vi "scope.vi"(7 "Channel Name":string="0" caption="Channel(s)", 8 "Trigger Type":T1(tab)=enum."Hysteresis", 9 "Min Sample Rate":dbl=10000.0 caption="Min. Sample Rate" step=1000000.0 format="%#.2p", 10 "error in":errorcluster, 11 "instrument handle":refnum<k15>) -> (0 "median":dbl=-0.00010879155888687819 format="%0.2f", 1 "Waveform(s)":waveform(dbl)(graph), 2 "error out":errorcluster, 3 "instrument handle out":refnum<k15>, 4 "low_level":dbl=-0.00010879155888687819, 6 "high_level":dbl=0.016276325847857098)   [LabVIEW 2018]
uses:
  <instrlib>/niScope/Configure/Trigger/niScope Configure Trigger Immediate.vi
  <instrlib>/niScope/Configure/Trigger/niScope Configure Trigger Edge.vi
  <instrlib>/niScope/Configure/Trigger/niScope Configure Trigger Digital.vi
  <instrlib>/niScope/Configure/Trigger/niScope Configure Trigger Window.vi
  <instrlib>/niScope/Configure/Trigger/niScope Configure Trigger Hysteresis.vi
  <instrlib>/niScope/Acquire/Fetch/niScope Fetch WDT.vi
  <vilib>/Analysis/NI_AALBase.lvlib
panel:
  in  "Trigger Source":string(combo)="0"
  in  "Trigger Level":dbl format="%.2f"
  in  "Trigger Slope":i32(ring) items=["Positive", "Negative"]
  in  "Coupling":u16(ring)=1 caption="Trigger Coupling" items=["AC"=0, "DC"=1, "HF Reject"=3, "LF Reject"=4, "AC Plus HF Reject"=1001]
  in  "Trigger Slope 2":i32(ring) caption="Trigger Slope" items=["Positive", "Negative"]
  in  "Trigger Source 2":string(combo)="VAL_PFI_1" caption="Trigger Source"
  in  "Coupling 2":u16(ring)=1 caption="Trigger Coupling" items=["AC"=0, "DC"=1, "HF Reject"=3, "LF Reject"=4, "AC Plus HF Reject"=1001]
  in  "High Level":dbl=0.1 caption="Window High Level" format="%.2f"
  in  "Low Level":dbl=-0.1 caption="Window Low Level" format="%.2f"
  in  "Window Mode":i32(ring) items=["Entering", "Leaving"]
  in  "Trigger Source 3":string(combo)="0" caption="Trigger Source"
  in  "Hysteresis":dbl=0.05 format="%.2f"
  in  "Trigger Source 4":string(combo)="0" caption="Trigger Source"
  in  "Trigger Level 2":dbl caption="Trigger Level" format="%.2f"
  in  "Coupling 3":u16(ring)=1 caption="Trigger Coupling" items=["AC"=0, "DC"=1, "HF Reject"=3, "LF Reject"=4, "AC Plus HF Reject"=1001]
  in  "Trigger Slope 3":i32(ring) caption="Trigger Slope" items=["Positive", "Negative"]
  out "Auto Triggered":bool=TRUE
  in  "Trigger Modifier":i32(ring)=2 items=["None"=1, "Auto Trigger"=2]
  in  "Vertical Coupling":i32(ring)=1 items=["AC", "DC", "Ground"]
  in  "Reference Position":dbl=50.0 caption="Ref Position" format="%.1f"
  in  "Trigger Delay":dbl caption="Trigger Delay (s)" format="%#.4p"
  in  "Maximum Input Frequency":dbl caption="Max. Input Frequency (Hz)" format="%.2f"
  in  "Input Impedance":u32(ring) items=["1 mega ohm"=0, "50 ohms"=2]
  in  "Probe Attenuation":dbl=1.0 format="%.1f"
  in  "Vertical Offset":dbl caption="Vertical Offset (V)" format="%.2p"
  in  "Timeout (s)":dbl=5.0 caption="Timeout(s)" format="%.2f"
  out "Actual Sample Rate":dbl=10000.0 format="%#.2p"
  out "Actual Record Length":i32=500
  in  "Min Record Length":i32=1000 caption="Min. Record Length"
  in  "Vertical Range":dbl=4.0 caption="Vertical Range (V)" format="%.2f"
  in  "Enforce Realtime":bool=TRUE
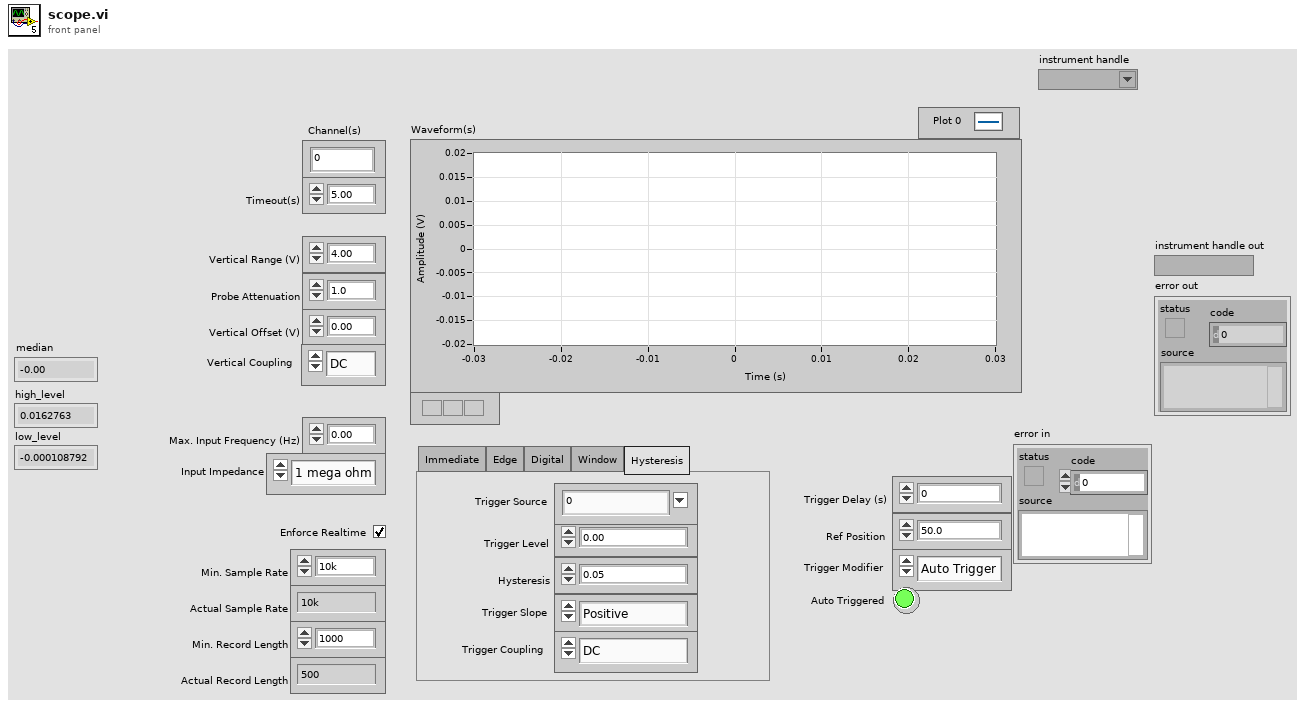
[diagram p1: front panel]
types:
  T1 = enum32{"Immediate", "Edge", "Digital", "Window", "Hysteresis"}
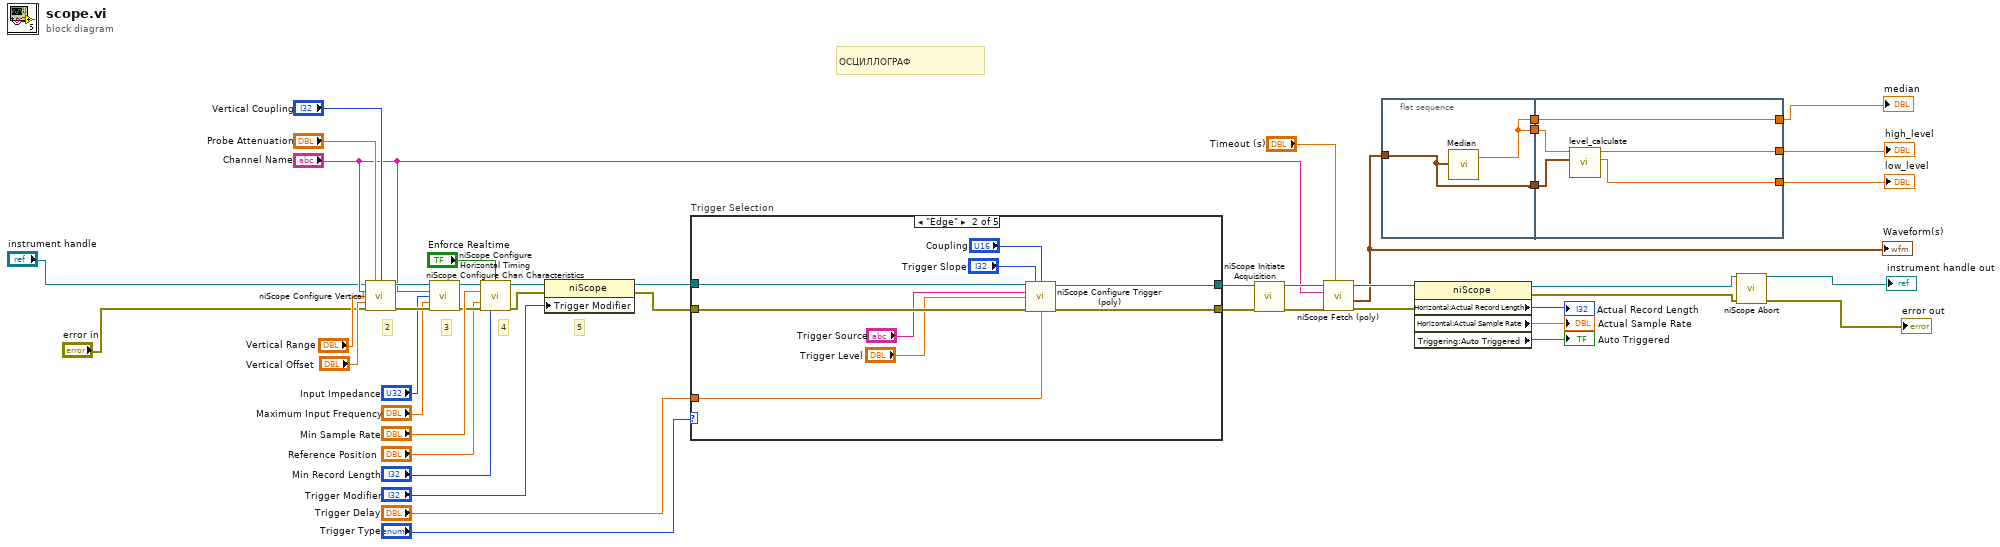
[diagram p0: block diagram]
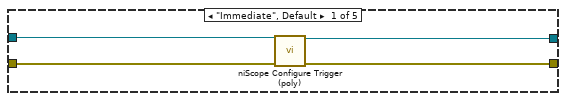
[diagram p2: hidden frame]
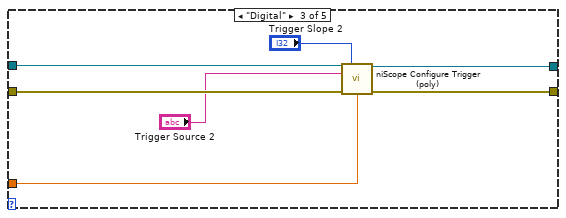
[diagram p3: hidden frame]
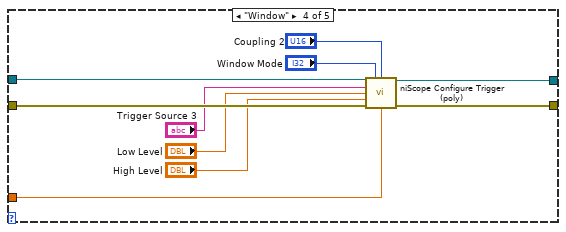
[diagram p4: hidden frame]
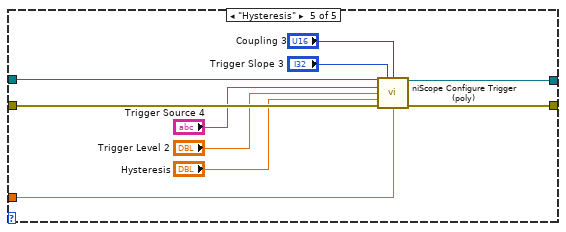
[diagram p5: hidden frame]
diagram:
  # "5"
  # "2"
  # "3"
  # "4"
  # "ОСЦИЛЛОГРАФ"
  n1 = call <instrlib>:"niScope Configure Vertical.vi"("instrument handle"="instrument handle", "probe attenuation"="Probe Attenuation", "vertical coupling"="Vertical Coupling", "channels"="Channel Name", "vertical range"="Vertical Range", "vertical offset"="Vertical Offset", "error in"="error in") -> ("instrument handle out"=w39:refnum<k15>, "error out"=w38:errorcluster)  [unwired: 7 in]
  n2 = call <instrlib>:"niScope Configure Chan Characteristics.vi"("instrument handle"=w39, "channels"="Channel Name", "input impedance"="Input Impedance", "maximum input frequency"="Maximum Input Frequency", "error in"=w38) -> ("instrument handle out"=w36:refnum<k15>, "error out"=w37:errorcluster)  [unwired: 9 in]
  n3 = call <instrlib>:"niScope Configure Horizontal Timing.vi"("instrument handle"=w36, "enforce realtime"="Enforce Realtime", "min sample rate"="Min Sample Rate", "reference position"="Reference Position", "error in"=w37, "min record length"="Min Record Length") -> ("instrument handle out"=w23:refnum<k15>, "error out"=w22:errorcluster)  [unwired: 8 in]
  n4 = property on="Property Node" class="niScope"(reference=w23, error in=w22, "Trigger Modifier"="Trigger Modifier") -> (reference out=w20:refnum<k15>, error out=w21:errorcluster)
  n5 = case "Trigger Selection" shown="\"Edge\"" "Trigger Type" {
    tunnel: w21 -> [w49 w58 w65 w75 w85]
    tunnel: [w46 w54 w61 w71 w81] -> w25
    tunnel: w20 -> [w48 w57 w64 w74 w84]
    tunnel: [w47 w55 w62 w72 w83] -> w28
    tunnel: "Trigger Delay" -> [_ w56 w63 w73 w82]
    frame "Immediate", Default {
      n6 = call-poly <instrlib>:"niScope Configure Trigger (poly).vi"("instrument handle"=w48, "error in"=w49) -> ("instrument handle out"=w47:refnum<k15>, "error out"=w46:errorcluster)  [unwired: 12 in]
    }
    frame "Edge" {
      n7 = call-poly <instrlib>:"niScope Configure Trigger (poly).vi"("instrument handle"=w57, "trigger slope"="Trigger Slope", "trigger coupling"="Coupling", "trigger source"="Trigger Source", "trigger level"="Trigger Level", "error in"=w58, "trigger delay"=w56) -> ("instrument handle out"=w55:refnum<k15>, "error out"=w54:errorcluster)  [unwired: 7 in]
    }
    frame "Digital" {
      n8 = call-poly <instrlib>:"niScope Configure Trigger (poly).vi"("instrument handle"=w64, "trigger slope"="Trigger Slope 2", "trigger source"="Trigger Source 2", "error in"=w65, "trigger delay"=w63) -> ("instrument handle out"=w62:refnum<k15>, "error out"=w61:errorcluster)  [unwired: 9 in]
    }
    frame "Window" {
      n9 = call-poly <instrlib>:"niScope Configure Trigger (poly).vi"("instrument handle"=w74, "trigger window mode"="Window Mode", "trigger coupling"="Coupling 2", "trigger source"="Trigger Source 3", "low level"="Low Level", "high level"="High Level", "error in"=w75, "trigger delay"=w73) -> ("instrument handle out"=w72:refnum<k15>, "error out"=w71:errorcluster)  [unwired: 6 in]
    }
    frame "Hysteresis" {
      n10 = call-poly <instrlib>:"niScope Configure Trigger (poly).vi"("instrument handle"=w84, "trigger slope"="Trigger Slope 3", "trigger coupling"="Coupling 3", "trigger source"="Trigger Source 4", "trigger level"="Trigger Level 2", "hysteresis"="Hysteresis", "error in"=w85, "trigger delay"=w82) -> ("instrument handle out"=w83:refnum<k15>, "error out"=w81:errorcluster)  [unwired: 6 in]
    }
  }
  n11 = call <instrlib>:"niScope Initiate Acquisition.vi"("instrument handle"=w28, "error in"=w25) -> ("instrument handle out"=w27:refnum<k15>, "error out"=w26:errorcluster)  [unwired: 12 in]
  n12 = call-poly <instrlib>:"niScope Fetch (poly).vi"("timeout"="Timeout (s)", "error in"=w26, "channels"="Channel Name", "instrument handle"=w27) -> ("error out"=w17:errorcluster, "wfm"=w10:waveform(dbl), "instrument handle out"=w18:refnum<k15>)  [unwired: 4 in, 1 out]
  "Waveform(s)" <- w10
  n13 = flat-sequence {
    tunnel: w10 -> [w86]
    tunnel: [w86] -> w45
    tunnel: [w87] -> w44
    tunnel: [w87] -> w43
    tunnel: w45 -> [w92]
    tunnel: w44 -> [w91]
    tunnel: [w90] -> w7
    tunnel: [w89] -> w6
    tunnel: [w88] -> w5
    tunnel: w43 -> [w88]
    frame #0 {
      n14 = call <vilib>:"Median.vi"("X"=w86) -> ("median"=w87:dbl)  [unwired: 1 out]
    }
    frame #1 {
      n15 = call "level_calculate.vi"("wfm"=w92, "y"=w91) -> ("low_level"=w90:dbl, "high_level"=w89:dbl)  [unwired: 8 in]
    }
  }
  n16 = property class="niScope"(reference=w18, error in=w17) -> (reference out=w8:refnum<k15>, error out=w9:errorcluster, "Horizontal:Actual Record Length"=→"Actual Record Length":i32, "Horizontal:Actual Sample Rate"=→"Actual Sample Rate":dbl, "Triggering:Auto Triggered"=→"Auto Triggered":bool)
  n17 = call <instrlib>:"niScope Abort.vi"("instrument handle"=w8, "error in"=w9) -> ("instrument handle out"=→"instrument handle out":refnum<k15>, "error out"=→"error out":errorcluster)  [unwired: 12 in]
  "high_level" <- w6
  "low_level" <- w7
  "median" <- w5
